vi "time-parse.vi"(8 "greatest ts diff":i32, 9 "ts least":timestamp, 10 "Array in":string[][](array[string]), 11 "type":u16(ring) caption="Relative Time Units" items=["SMART", "Seconds", "Minutes", "Hours", "All"]) -> (2 "Array out":string[][](array[string]))   [LabVIEW 2017]
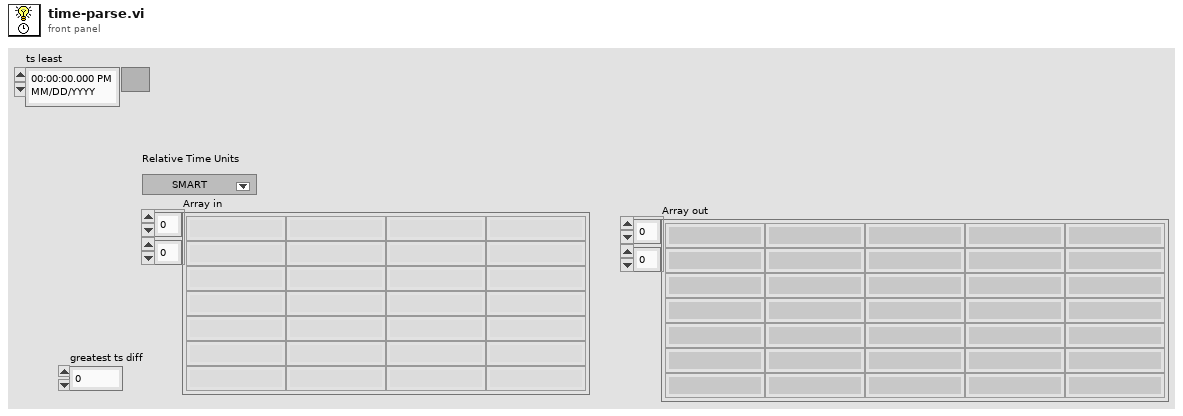
[diagram p1: front panel]
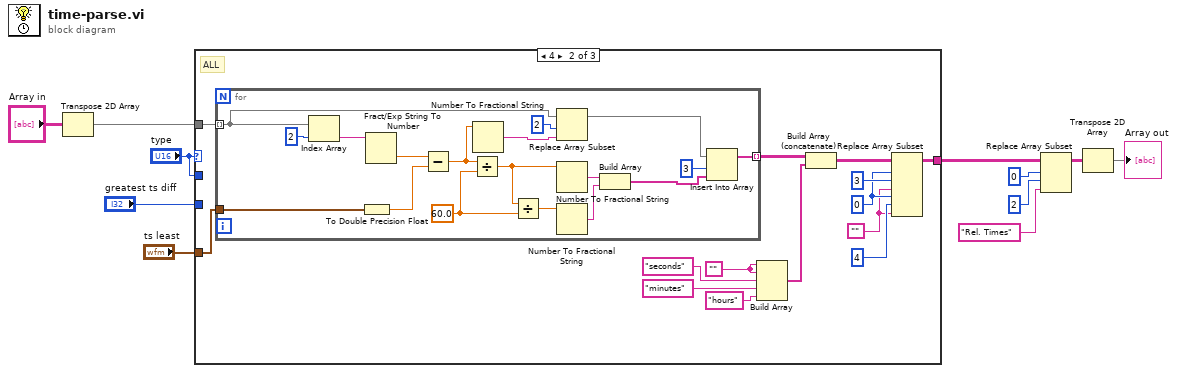
[diagram p0: block diagram]
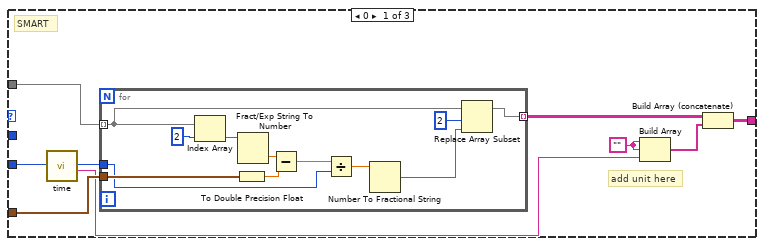
[diagram p2: hidden frame]
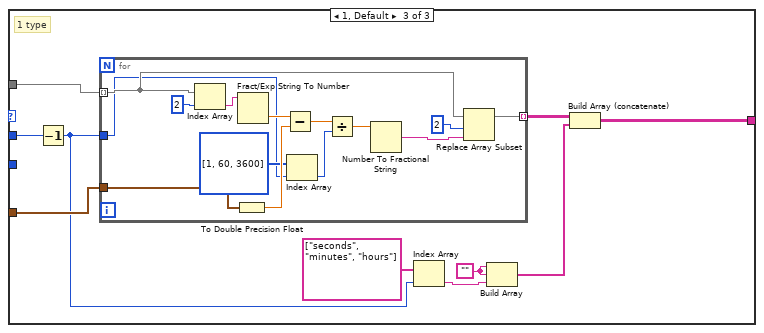
[diagram p3: hidden frame]
diagram:
  n1 = Transpose 2D Array(2D array="Array in") -> (transposed array=w11:string[][])
  n2 = case shown="4" "type" {
    tunnel: w11 -> [w15 w45 w73]
    tunnel: [w13 w33 w66] -> w2
    tunnel: "greatest ts diff" -> [w20 _ _]
    tunnel: "ts least" -> [w18 w44 w72]
    tunnel: "type" -> [_ _ w68]
    frame 0 {
      w16 = ""
      # "add unit here"
      # "SMART"
      n3 = call "time.vi"("# seconds"=w20) -> ("unit"=w17:string, "reduction"=w19:i32)  [unwired: 7 in, 1 out]
      n4 = for {
        tunnel: w15 -> [w31] mode=indexing
        tunnel: [w30] -> w12 mode=indexing
        tunnel: w19 -> [w26]
        tunnel: w18 -> [w28]
        n5 = Index Array(array=w31, index=2) -> (element=w22:string)
        n6 = To Double Precision Float(number=w28) -> (double precision float=w23:dbl)
        n7 = Fract/Exp String To Number(string=w22) -> (number=w21:dbl)  [unwired: 3 in, 1 out]
        n8 = Subtract(x=w21, y=w23) -> (x-y=w27:dbl)
        n9 = Divide(x=w27, y=w26) -> (x/y=w24:dbl)
        n10 = Number To Fractional String(number=w24) -> (F-format string=w25:string)  [unwired: 3 in]
        n11 = Replace Array Subset(array=w31, new element=w25, index=2) -> (w30:string[])
      }
      n12 = Build Array(w16, w16, w17) -> (w14:string[])
      n13 = Build Array (concatenate)(w12, w14) -> (w13:string[][])
    }
    frame 4 {
      w34 = ""
      w36 = 0 ("index (row)")
      w46 = ""
      # "ALL"
      n14 = for {
        tunnel: w45 -> [w51] mode=indexing
        tunnel: [w53] -> w40 mode=indexing
        tunnel: w44 -> [w60]
        w56 = 60.0 ("y")
        n15 = Index Array(array=w51, index=2) -> (element=w63:string)
        n16 = To Double Precision Float(number=w60) -> (double precision float=w61:dbl)
        n17 = Fract/Exp String To Number(string=w63) -> (number=w62:dbl)  [unwired: 3 in, 1 out]
        n18 = Subtract(x=w62, y=w61) -> (x-y=w59:dbl)
        n19 = Divide(x=w59, y=w56) -> (x/y=w57:dbl)
        n20 = Number To Fractional String(number=w59) -> (F-format string=w50:string)  [unwired: 3 in]
        n21 = Divide(x=w57, y=w56) -> (x/y=w55:dbl)
        n22 = Replace Array Subset(array=w51, new element=w50, index=2) -> (w48:string[])
        n23 = Number To Fractional String(number=w57) -> (F-format string=w58:string)  [unwired: 3 in]
        n24 = Number To Fractional String(number=w55) -> (F-format string=w54:string)  [unwired: 3 in]
        n25 = Build Array(w58, w54) -> (w52:string[])
        n26 = Insert Into Array(array=w48, index=3, new element=w52) -> (w53:string[])
      }
      n27 = Build Array(w46, w46, "seconds" ("element"), "minutes" ("element"), "hours" ("element")) -> (w39:string[])
      n28 = Build Array (concatenate)(w40, w39) -> (w38:string[][])
      n29 = Replace Array Subset(array=w38, new element #1=w34, index (row) #1=w36, index (col) #1=3 ("disabled index (col)"), new element #2=w34, index (row) #2=w36, index (col) #2=4 ("disabled index (col)")) -> (w33:string[][])
    }
    frame 1, Default {
      w74 = ""
      # "1 type"
      n30 = Decrement(x=w68) -> (x-1=w70:u16)
      n31 = for {
        tunnel: w73 -> [w87] mode=indexing
        tunnel: [w86] -> w65 mode=indexing
        tunnel: w72 -> [w81]
        tunnel: w70 -> [w76]
        n32 = Index Array(array=w87, index=2) -> (element=w84:string)
        n33 = To Double Precision Float(number=w81) -> (double precision float=w82:dbl)
        n34 = Fract/Exp String To Number(string=w84) -> (number=w83:dbl)  [unwired: 3 in, 1 out]
        n35 = Subtract(x=w83, y=w82) -> (x-y=w80:dbl)
        n36 = Index Array(array=i32[] [1, 60, 3600], index=w76) -> (element=w75:i32)
        n37 = Divide(x=w80, y=w75) -> (x/y=w78:dbl)
        n38 = Number To Fractional String(number=w78) -> (F-format string=w79:string)  [unwired: 3 in]
        n39 = Replace Array Subset(array=w87, new element=w79, index=2) -> (w86:string[])
      }
      n40 = Index Array(array=string[] ["seconds", "minutes", "hours"], index=w70) -> (element=w69:string)
      n41 = Build Array(w74, w74, w69) -> (w67:string[])
      n42 = Build Array (concatenate)(w65, w67) -> (w66:string[][])
    }
  }
  n43 = Replace Array Subset(array=w2, new element="Rel. Times", index (row)=0, index (col)=2 ("disabled index (col)")) -> (w1:string[][])
  n44 = Transpose 2D Array(2D array=w1) -> (transposed array=→"Array out":string[][])
